vi "Get Default Overload Prot Tmo.vi"(8 "error in (no error)":errorcluster, 11 "VISA resource name":refnum<visa-resource-name>) -> (0 "error out":errorcluster, 2 "Default Timeout Value":dbl format="%.4f", 3 "VISA resource name out":refnum<visa-resource-name>)   [LabVIEW 2013, in "Fluke 5XXX Series Multicalibrators.lvlib"]
doc: "This VI returns the programmed default OPERATE time limit for the OVERLD mode signal.\n\nNote:\n\nThis VI is available only for instrument models 5500A and 5520A with oscilloscope option SC600 (SC1100)."
uses:
  Fluke 5XXX Series Multicalibrators.lvlib
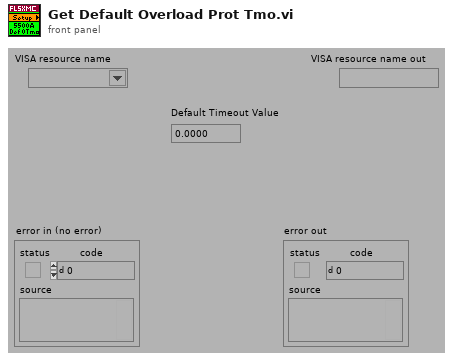
[diagram p1: front panel]
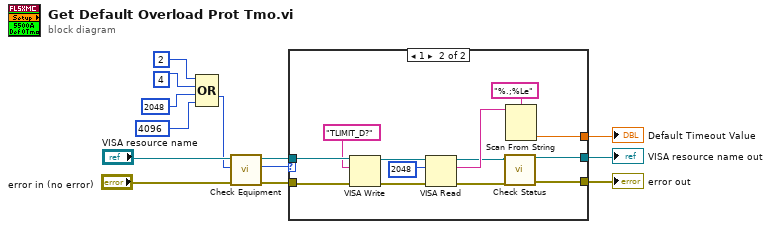
[diagram p0: block diagram]
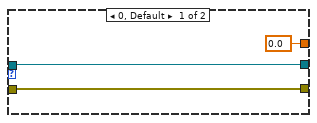
[diagram p2: hidden frame]
diagram:
  n1 = Compound Arithmetic op=OR(2 ("Numeric"), 4 ("Numeric"), 2048 ("Numeric"), 4096 ("Numeric")) -> (w2:i32)
  n2 = call "Check Equipment.vi"("error in (no error)"="error in (no error)", "Bit Mask"=w2, "VISA resource name"="VISA resource name") -> ("error out"=w9:errorcluster, "Present?"=w8:u32, "VISA resource name out"=w7:refnum<visa-resource-name>)  [unwired: 6 in]
  n3 = case shown="1" w8 {
    tunnel: w9 -> [w16 w28]
    tunnel: w7 -> [w14 w27]
    tunnel: [w16 w29] -> w6
    tunnel: [0.0 w18] -> w5
    tunnel: [w14 w17] -> w1
    frame 0, Default {
    }
    frame 1 {
      n4 = VISA Write(VISA resource name=w27, write buffer="TLIMIT_D?", error in (no error)=w28) -> (VISA resource name out=w24:refnum<visa-resource-name>, error out=w23:errorcluster)  [unwired: 1 out]
      n5 = VISA Read(VISA resource name=w24, byte count=u32 2048 ("byte count (0)"), error in (no error)=w23) -> (VISA resource name out=w19:refnum<visa-resource-name>, read buffer=w20:string, error out=w21:errorcluster)  [unwired: 1 out]
      n6 = call "Check Status.vi"("VISA resource name"=w19, "error in (no error)"=w21) -> ("VISA resource name out"=w17:refnum<visa-resource-name>, "error out"=w29:errorcluster)  [unwired: 12 in]
      n7 = Scan From String(format string="%.;%Le", input string=w20) -> (output 1=w18:dbl)  [unwired: 3 in, 3 out]
    }
  }
  "Default Timeout Value" <- w5
  "VISA resource name out" <- w1
  "error out" <- w6
